vi "PCSMain.get Objects on same node.vi"(0 "i ref in":refnum<vi>, 5 "error in (no error)":errorcluster) -> (14 "i ref out":refnum<vi>, 19 "error out":errorcluster)   [LabVIEW 2014, in "PCSMain.lvlib"]
doc: "This VI gets all objects running at the same node."
uses:
  PCSMain.lvlib
  CS_Core/CSSystem/CSSystemLib/CSSystemLib.lvlib
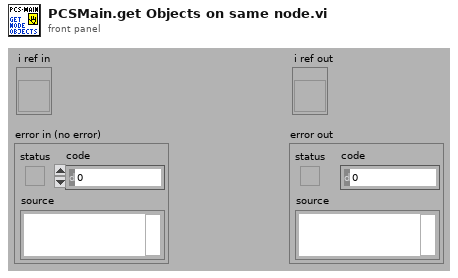
[diagram p1: front panel]
types:
  T1 = typedef "PCSMain.lvlib/PCSMain.i attribute.ctl" = cluster{"System Objects":cluster{"Spectrometer Objects":string[], "Camera Objects":string[], "Image Operator Objects":string[], "Gate- and Delaygenerators":string[], "Current Meas Objects":string[], "Calorimeter Objects":string[], "Powermeter Objects":string[], "SSAC Objects":string[], "Vacuum Control Objects":string[], "Countdown Counter Objects":string[], "Beckhoff Watchdog Objects":string[], "SHS Analyzer Objects":string[]}, "Local Objects":cluster{"Spectrometer Objects":string[], "Camera Objects":string[], "Image Operator Objects":string[], "Gate- and Delaygenerators":string[], "Current Meas Objects":string[], "Calorimeter Objects":string[], "Powermeter Objects":string[], "SSAC Objects":string[], "Vacuum Control Objects":string[], "Countdown Counter Objects":string[], "Beckhoff Watchdog Objects":string[], "SHS Analyzer Objects":string[]}, "Systems on same node":string[], "Data Viewer visible?":bool, "Running Objects":cluster{"Operators":bool, "SHS Analyzers":bool}, "Cam Instance System ID":string, "Black Box Objects":string[], "Switch Objects":string[], "Motion GUI Objects":string[], "Osci Objects":string[]}
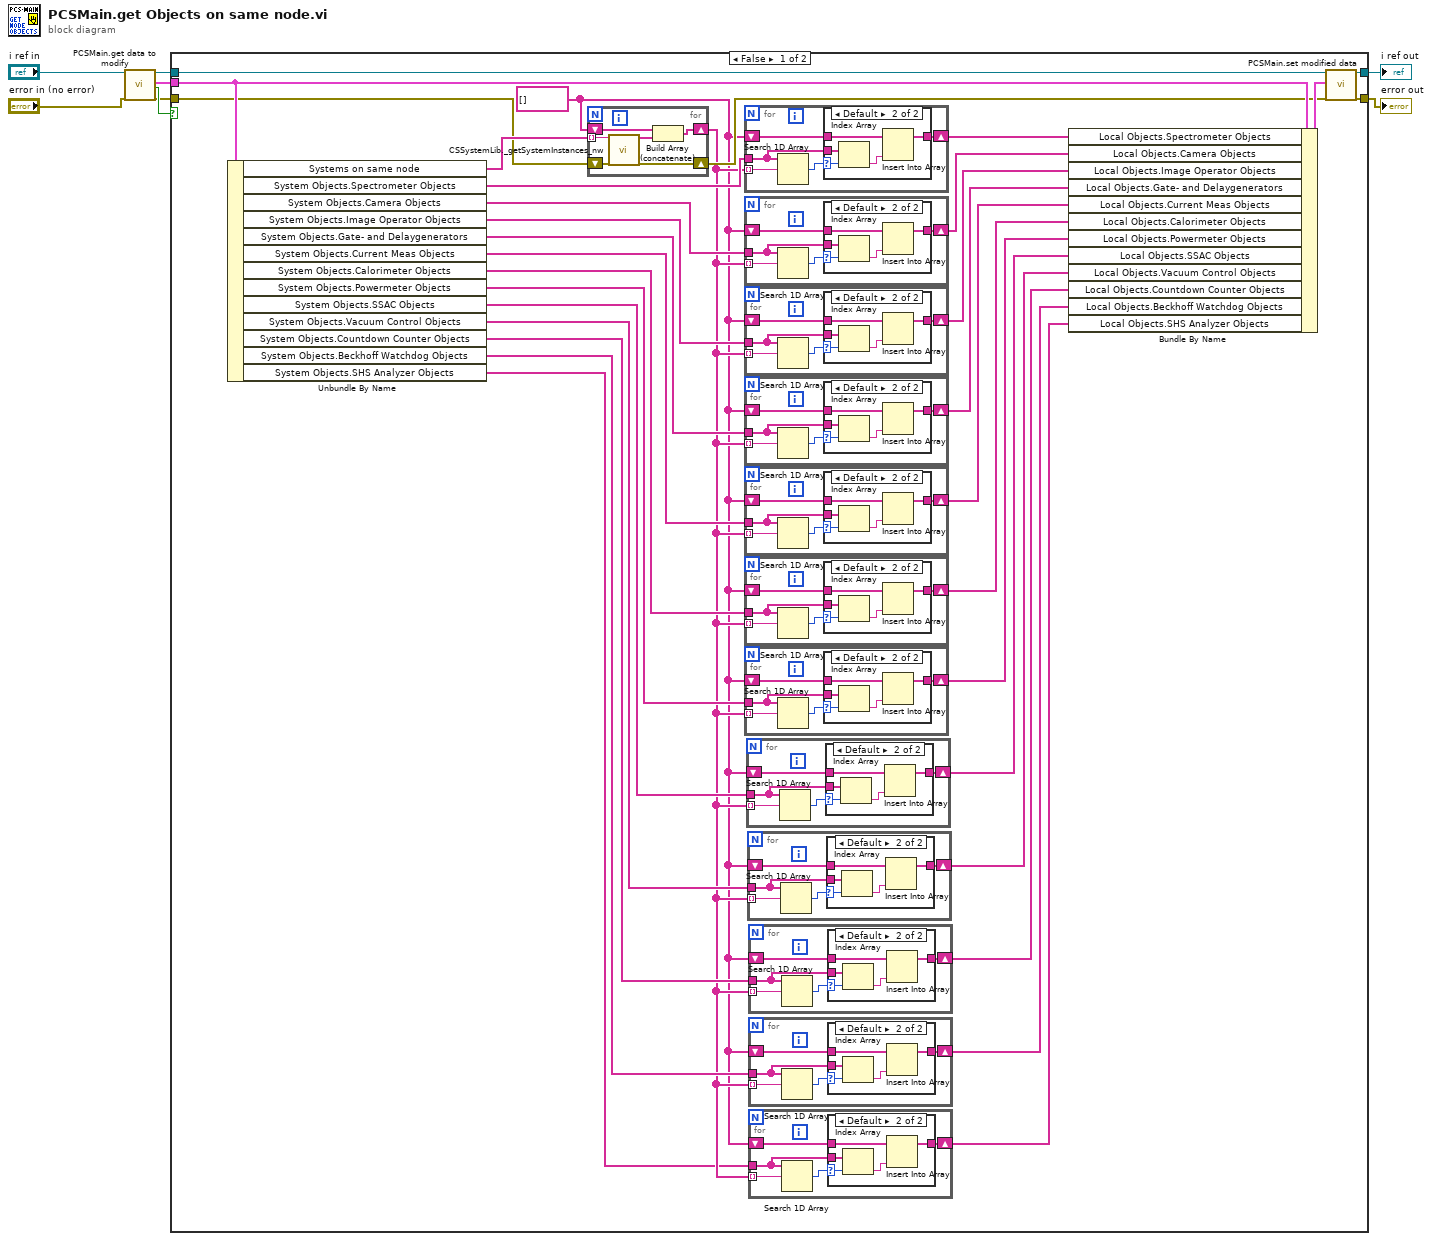
[diagram p0: block diagram]
diagram:
  n1 = call "PCSMain.get data to modify.vi"("i ref in"="i ref in", "error in (no error)"="error in (no error)") -> ("i ref out"=w1:refnum<vi>, "i attribute"=w4:T1, "timed out"=w3:bool, "error out"=w2:errorcluster)  [unwired: 14 in]
  n2 = case shown="False" w3 {
    tunnel: w1 -> [w42 w182]
    tunnel: [w41 w182] -> w5
    tunnel: w2 -> [w22 w181]
    tunnel: [w40 w181] -> w6
    tunnel: w4 -> [w39 _]
    frame False {
      w10 = string[] []
      n3 = Unbundle By Name(w39) -> ("Systems on same node"=w23:string[], "System Objects.Spectrometer Objects"=w38:string[], "System Objects.Camera Objects"=w36:string[], "System Objects.Image Operator Objects"=w35:string[], "System Objects.Gate- and Delaygenerators"=w34:string[], "System Objects.Current Meas Objects"=w33:string[], "System Objects.Calorimeter Objects"=w32:string[], "System Objects.Powermeter Objects"=w31:string[], "System Objects.SSAC Objects"=w20:string[], "System Objects.Vacuum Control Objects"=w18:string[], "System Objects.Countdown Counter Objects"=w16:string[], "System Objects.Beckhoff Watchdog Objects"=w13:string[], "System Objects.SHS Analyzer Objects"=w9:string[])
      n4 = for {
        tunnel: w23 -> [w103] mode=indexing
        shift-right: [w101] -> w12
        shift-left: w10 -> [w100]
        shift-right: [w98] -> w21
        shift-left: w22 -> [w99]
        n5 = call "CSSystemLib._getSystemInstances_nw.vi"("systemName"=w103, "error in (no error)"=w99) -> ("i list"=w102:string[], "error out"=w98:errorcluster)  [unwired: 16 in]
        n6 = Build Array (concatenate)(w100, w102) -> (w101:string[])
      }
      n7 = for {
        tunnel: w38 -> [w173]
        tunnel: w12 -> [w174] mode=indexing
        shift-right: [w172] -> w25
        shift-left: w10 -> [w171]
        n8 = Search 1D Array(1D array=w173, element=w174) -> (index of element=w170:i32)  [unwired: 1 in]
        n9 = case shown="Default" w170 {
          selector: w170 -> [_ w176]
          tunnel: w173 -> [_ w180]
          tunnel: [w175 w178] -> w172
          tunnel: w171 -> [w175 w177]
          frame -1 {
          }
          frame Default {
            n10 = Index Array(array=w180, index=w176) -> (element=w179:string)
            n11 = Insert Into Array(array=w177, new element=w179) -> (w178:string[])  [unwired: 1 in]
          }
        }
      }
      n12 = for {
        tunnel: w36 -> [w162]
        tunnel: w12 -> [w163] mode=indexing
        shift-right: [w161] -> w24
        shift-left: w10 -> [w160]
        n13 = Search 1D Array(1D array=w162, element=w163) -> (index of element=w159:i32)  [unwired: 1 in]
        n14 = case shown="Default" w159 {
          selector: w159 -> [_ w165]
          tunnel: w162 -> [_ w169]
          tunnel: [w164 w167] -> w161
          tunnel: w160 -> [w164 w166]
          frame -1 {
          }
          frame Default {
            n15 = Index Array(array=w169, index=w165) -> (element=w168:string)
            n16 = Insert Into Array(array=w166, new element=w168) -> (w167:string[])  [unwired: 1 in]
          }
        }
      }
      n17 = for {
        tunnel: w35 -> [w151]
        tunnel: w12 -> [w152] mode=indexing
        shift-right: [w150] -> w30
        shift-left: w10 -> [w149]
        n18 = Search 1D Array(1D array=w151, element=w152) -> (index of element=w148:i32)  [unwired: 1 in]
        n19 = case shown="Default" w148 {
          selector: w148 -> [_ w154]
          tunnel: w151 -> [_ w158]
          tunnel: [w153 w156] -> w150
          tunnel: w149 -> [w153 w155]
          frame -1 {
          }
          frame Default {
            n20 = Index Array(array=w158, index=w154) -> (element=w157:string)
            n21 = Insert Into Array(array=w155, new element=w157) -> (w156:string[])  [unwired: 1 in]
          }
        }
      }
      n22 = for {
        tunnel: w34 -> [w118]
        tunnel: w12 -> [w119] mode=indexing
        shift-right: [w117] -> w29
        shift-left: w10 -> [w116]
        n23 = Search 1D Array(1D array=w118, element=w119) -> (index of element=w115:i32)  [unwired: 1 in]
        n24 = case shown="Default" w115 {
          selector: w115 -> [_ w121]
          tunnel: w118 -> [_ w125]
          tunnel: [w120 w123] -> w117
          tunnel: w116 -> [w120 w122]
          frame -1 {
          }
          frame Default {
            n25 = Index Array(array=w125, index=w121) -> (element=w124:string)
            n26 = Insert Into Array(array=w122, new element=w124) -> (w123:string[])  [unwired: 1 in]
          }
        }
      }
      n27 = for {
        tunnel: w33 -> [w140]
        tunnel: w12 -> [w141] mode=indexing
        shift-right: [w139] -> w28
        shift-left: w10 -> [w138]
        n28 = Search 1D Array(1D array=w140, element=w141) -> (index of element=w137:i32)  [unwired: 1 in]
        n29 = case shown="Default" w137 {
          selector: w137 -> [_ w143]
          tunnel: w140 -> [_ w147]
          tunnel: [w142 w145] -> w139
          tunnel: w138 -> [w142 w144]
          frame -1 {
          }
          frame Default {
            n30 = Index Array(array=w147, index=w143) -> (element=w146:string)
            n31 = Insert Into Array(array=w144, new element=w146) -> (w145:string[])  [unwired: 1 in]
          }
        }
      }
      n32 = for {
        tunnel: w32 -> [w107]
        tunnel: w12 -> [w108] mode=indexing
        shift-right: [w106] -> w27
        shift-left: w10 -> [w105]
        n33 = Search 1D Array(1D array=w107, element=w108) -> (index of element=w104:i32)  [unwired: 1 in]
        n34 = case shown="Default" w104 {
          selector: w104 -> [_ w110]
          tunnel: w107 -> [_ w114]
          tunnel: [w109 w112] -> w106
          tunnel: w105 -> [w109 w111]
          frame -1 {
          }
          frame Default {
            n35 = Index Array(array=w114, index=w110) -> (element=w113:string)
            n36 = Insert Into Array(array=w111, new element=w113) -> (w112:string[])  [unwired: 1 in]
          }
        }
      }
      n37 = for {
        tunnel: w31 -> [w129]
        tunnel: w12 -> [w130] mode=indexing
        shift-right: [w128] -> w26
        shift-left: w10 -> [w127]
        n38 = Search 1D Array(1D array=w129, element=w130) -> (index of element=w126:i32)  [unwired: 1 in]
        n39 = case shown="Default" w126 {
          selector: w126 -> [_ w132]
          tunnel: w129 -> [_ w136]
          tunnel: [w131 w134] -> w128
          tunnel: w127 -> [w131 w133]
          frame -1 {
          }
          frame Default {
            n40 = Index Array(array=w136, index=w132) -> (element=w135:string)
            n41 = Insert Into Array(array=w133, new element=w135) -> (w134:string[])  [unwired: 1 in]
          }
        }
      }
      n42 = for {
        tunnel: w20 -> [w90]
        tunnel: w12 -> [w91] mode=indexing
        shift-right: [w89] -> w19
        shift-left: w10 -> [w88]
        n43 = Search 1D Array(1D array=w90, element=w91) -> (index of element=w87:i32)  [unwired: 1 in]
        n44 = case shown="Default" w87 {
          selector: w87 -> [_ w93]
          tunnel: w90 -> [_ w97]
          tunnel: [w92 w95] -> w89
          tunnel: w88 -> [w92 w94]
          frame -1 {
          }
          frame Default {
            n45 = Index Array(array=w97, index=w93) -> (element=w96:string)
            n46 = Insert Into Array(array=w94, new element=w96) -> (w95:string[])  [unwired: 1 in]
          }
        }
      }
      n47 = for {
        tunnel: w18 -> [w79]
        tunnel: w12 -> [w80] mode=indexing
        shift-right: [w78] -> w17
        shift-left: w10 -> [w77]
        n48 = Search 1D Array(1D array=w79, element=w80) -> (index of element=w76:i32)  [unwired: 1 in]
        n49 = case shown="Default" w76 {
          selector: w76 -> [_ w82]
          tunnel: w79 -> [_ w86]
          tunnel: [w81 w84] -> w78
          tunnel: w77 -> [w81 w83]
          frame -1 {
          }
          frame Default {
            n50 = Index Array(array=w86, index=w82) -> (element=w85:string)
            n51 = Insert Into Array(array=w83, new element=w85) -> (w84:string[])  [unwired: 1 in]
          }
        }
      }
      n52 = for {
        tunnel: w16 -> [w68]
        tunnel: w12 -> [w69] mode=indexing
        shift-right: [w67] -> w15
        shift-left: w10 -> [w66]
        n53 = Search 1D Array(1D array=w68, element=w69) -> (index of element=w65:i32)  [unwired: 1 in]
        n54 = case shown="Default" w65 {
          selector: w65 -> [_ w71]
          tunnel: w68 -> [_ w75]
          tunnel: [w70 w73] -> w67
          tunnel: w66 -> [w70 w72]
          frame -1 {
          }
          frame Default {
            n55 = Index Array(array=w75, index=w71) -> (element=w74:string)
            n56 = Insert Into Array(array=w72, new element=w74) -> (w73:string[])  [unwired: 1 in]
          }
        }
      }
      n57 = for {
        tunnel: w13 -> [w57]
        tunnel: w12 -> [w58] mode=indexing
        shift-right: [w56] -> w14
        shift-left: w10 -> [w55]
        n58 = Search 1D Array(1D array=w57, element=w58) -> (index of element=w54:i32)  [unwired: 1 in]
        n59 = case shown="Default" w54 {
          selector: w54 -> [_ w60]
          tunnel: w57 -> [_ w64]
          tunnel: [w59 w62] -> w56
          tunnel: w55 -> [w59 w61]
          frame -1 {
          }
          frame Default {
            n60 = Index Array(array=w64, index=w60) -> (element=w63:string)
            n61 = Insert Into Array(array=w61, new element=w63) -> (w62:string[])  [unwired: 1 in]
          }
        }
      }
      n62 = for {
        tunnel: w9 -> [w46]
        tunnel: w12 -> [w47] mode=indexing
        shift-right: [w45] -> w11
        shift-left: w10 -> [w44]
        n63 = Search 1D Array(1D array=w46, element=w47) -> (index of element=w43:i32)  [unwired: 1 in]
        n64 = case shown="Default" w43 {
          selector: w43 -> [_ w49]
          tunnel: w46 -> [_ w53]
          tunnel: [w48 w51] -> w45
          tunnel: w44 -> [w48 w50]
          frame -1 {
          }
          frame Default {
            n65 = Index Array(array=w53, index=w49) -> (element=w52:string)
            n66 = Insert Into Array(array=w50, new element=w52) -> (w51:string[])  [unwired: 1 in]
          }
        }
      }
      n67 = Bundle By Name(cluster=w39, "Local Objects.Spectrometer Objects"=w25, "Local Objects.Camera Objects"=w24, "Local Objects.Image Operator Objects"=w30, "Local Objects.Gate- and Delaygenerators"=w29, "Local Objects.Current Meas Objects"=w28, "Local Objects.Calorimeter Objects"=w27, "Local Objects.Powermeter Objects"=w26, "Local Objects.SSAC Objects"=w19, "Local Objects.Vacuum Control Objects"=w17, "Local Objects.Countdown Counter Objects"=w15, "Local Objects.Beckhoff Watchdog Objects"=w14, "Local Objects.SHS Analyzer Objects"=w11) -> (w37:T1)
      n68 = call "PCSMain.set modified data.vi"("i ref in"=w42, "i attribute"=w37, "error in (no error)"=w21) -> ("i ref out"=w41:refnum<vi>, "error out"=w40:errorcluster)  [unwired: 15 in]
    }
    frame True {
    }
  }
  "error out" <- w6
  "i ref out" <- w5
